vi "Dispose ToolStrip Seperator.vi"(8 "error in (no error)":errorcluster caption="错误输入（无错误）", 11 "ToolsStripSeperator 输入":refnum<class "ToolsStripSeperator.lvclass"> caption="DNL_LabVIEW Object in") -> (0 "error out":errorcluster caption="错误输出", 3 "ToolsStripSeperator 输出":refnum<class "ToolsStripSeperator.lvclass"> caption="DNL_LabVIEW Object out")   [LabVIEW 2013, in "ToolsStripSeperator.lvclass"]
uses:
  ToolsStripSeperator.lvclass
  ToolsStripSeperator.lvclass/ToolsStripSeperator.ctl
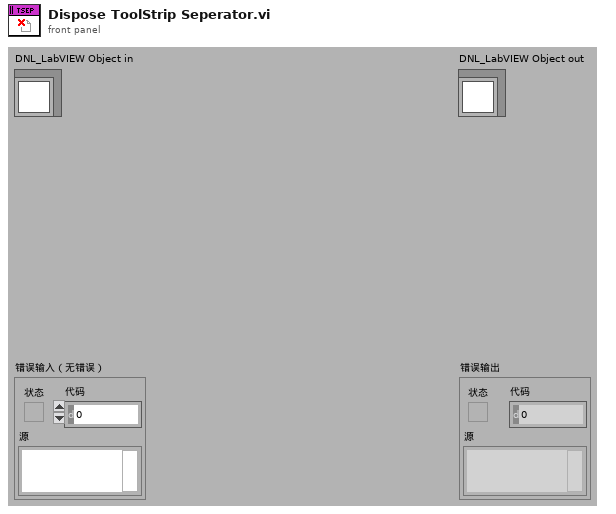
[diagram p1: front panel]
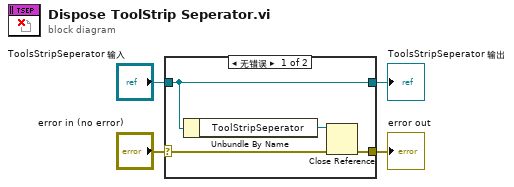
[diagram p0: block diagram]
diagram:
  n1 = case shown="无错误" "error in (no error)" {
    selector: "error in (no error)" -> [w6 w10]
    tunnel: [w5 w10] -> w3
    tunnel: [w8 w9] -> w1
    tunnel: "ToolsStripSeperator 输入" -> [w8 w9]
    frame No Error {
      n2 = Unbundle By Name(w8) -> ("ToolStripSeperator"=w7:refnum<k24>)
      n3 = Close Reference(reference=w7, error in (no error)=w6) -> (error out=w5:errorcluster)
    }
    frame Error {
    }
  }
  "error out" <- w3
  "ToolsStripSeperator 输出" <- w1
